vi "Add PV (DBL).vi"(5 "is read only? (F)":bool, 6 "initial timestamp":timestamp, 7 "PV name":string, 8 "error in (no error)":errorcluster, 9 "fields":T1, 10 "initial value":dbl format="%#_13g", 11 "Server in":refnum<class "Server.lvclass">) -> (0 "error out":errorcluster, 2 "value out":dbl, 3 "Server out":refnum<class "Server.lvclass">, 4 "timestamp out":timestamp)   [LabVIEW 2020, in "PV Access.lvlib" / "PVA Server.lvlib" / "Server.lvclass"]
uses:
  Server.lvclass
  PV Data/NT Scalar (Numeric)/NT Scalar (Numeric).lvclass
  C:/Users/eyw68381/source/repos/pvaccess-labview/labview/source/PV Data/NT Base/NT Base.lvclass
  Server.lvclass/Server.ctl
  Source/Source.lvclass
  PV Data/PV Data.lvlib
  PV Data/NT Scalar (Numeric)/Create (DBL).vi
  PV Data/Value Fields.ctl
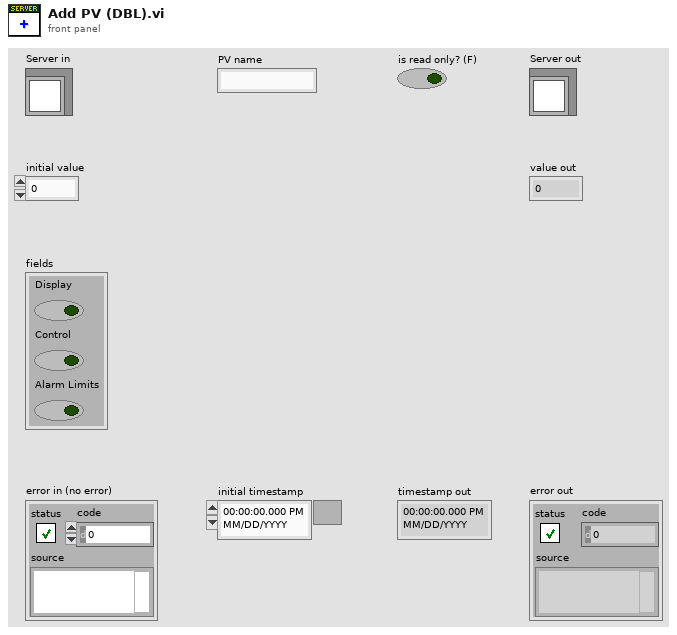
[diagram p1: front panel]
types:
  T1 = typedef "PV Access.lvlib/PV Data.lvlib/Value Fields.ctl" = cluster{"Display":bool, "Control":bool, "Alarm Limits":bool}
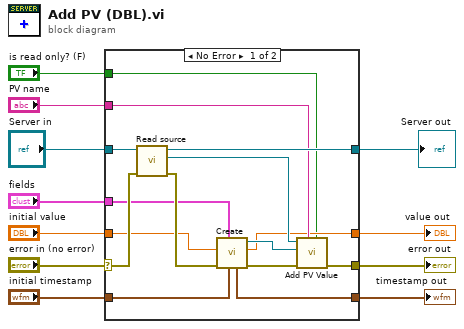
[diagram p0: block diagram]
diagram:
  n1 = case shown="No Error" "error in (no error)" {
    selector: "error in (no error)" -> [w22 w30]
    tunnel: [w21 w30] -> w10
    tunnel: [w25 w29] -> w8
    tunnel: "Server in" -> [w26 w29]
    tunnel: "PV name" -> [w23 _]
    tunnel: "initial value" -> [w17 w28]
    tunnel: [w16 w28] -> w5
    tunnel: "fields" -> [w15 _]
    tunnel: "initial timestamp" -> [w14 w27]
    tunnel: [w13 w27] -> w2
    tunnel: "is read only? (F)" -> [w12 _]
    frame No Error {
      n2 = call "Read source.vi"("error in (no error)"=w22, "Server in"=w26) -> ("error out"=w20:errorcluster, "Source"=w24:refnum<class "Source.lvclass">, "Server out"=w25:refnum<class "Server.lvclass">)  [unwired: 7 in]
      n3 = call-poly "Create.vi"("timestamp in"=w14, "fields"=w15, "error in (no error)"=w20, "value in"=w17) -> ("error out"=w19:errorcluster, "value out"=w16:dbl, "NT Scalar (Numeric) out"=w18:refnum<class "NT Scalar (Numeric).lvclass">, "timestamp out"=w13:timestamp)  [unwired: 4 in]
      n4 = call "Add PV Value.vi"("is read only? (F)"=w12, "PV name"=w23, "error in"=w19, "NT Base in"=w18, "Source in"=w24) -> ("error out"=w21:errorcluster)  [unwired: 4 in, 2 out]
    }
    frame Error {
    }
  }
  "error out" <- w10
  "Server out" <- w8
  "value out" <- w5
  "timestamp out" <- w2
